vi "Parse RW.vi"(8 "error in (no error)":errorcluster, 11 "R/W mode in":string) -> (0 "error out":errorcluster, 3 "R/W?":T1)   [LabVIEW 2018, in "Config_Read_BML.lvclass"]
uses:
  Config_Read_BML.lvclass
  RW_Option.ctl
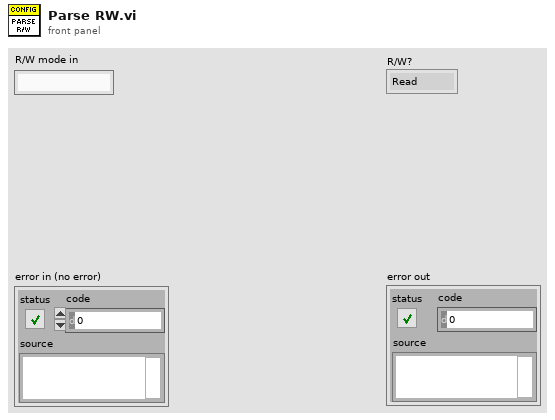
[diagram p1: front panel]
types:
  T1 = typedef "Config_Read_BML.lvclass/RW_Option.ctl" = enum16{"Read", "Write", "R/W"}
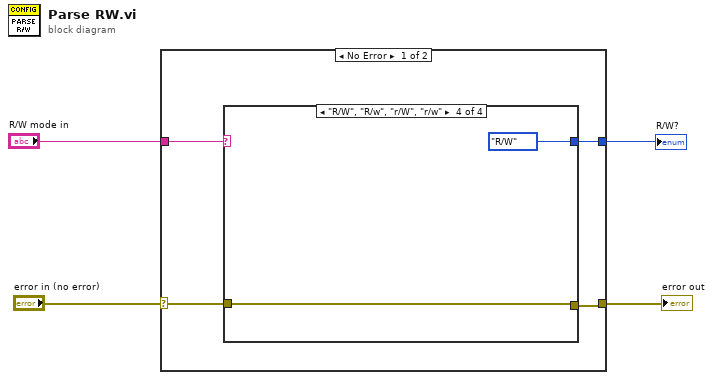
[diagram p0: block diagram]
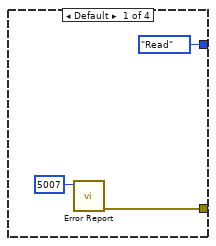
[diagram p2: hidden frame]
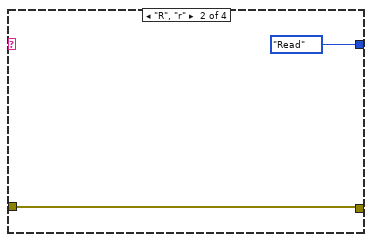
[diagram p3: hidden frame]
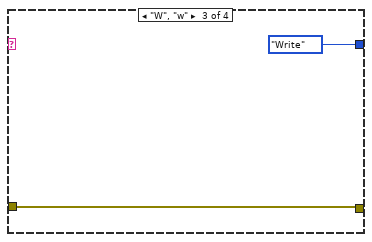
[diagram p4: hidden frame]
diagram:
  n1 = case shown="No Error" "error in (no error)" {
    selector: "error in (no error)" -> [w5 w18]
    tunnel: "R/W mode in" -> [w8 _]
    tunnel: [w6 w18] -> w2
    tunnel: [w7 _] -> w1
    frame No Error {
      n2 = case shown="\"R/W\", \"R/w\", \"r/W\", \"r/w\"" w8 {
        tunnel: [RW_Option."Read" ("R/W?") RW_Option."Read" ("R/W?") RW_Option."Write" ("R/W?") RW_Option."R/W" ("R/W?")] -> w7
        tunnel: [w10 w12 w14 w16] -> w6
        tunnel: w5 -> [_ w12 w14 w16]
        frame Default {
          n3 = call "Error Report.vi"("Error Code"=i16 5007) -> ("error out"=w10:errorcluster)  [unwired: 10 in]
        }
        frame "R", "r" {
        }
        frame "W", "w" {
        }
        frame "R/W", "R/w", "r/W", "r/w" {
        }
      }
    }
    frame Error {
    }
  }
  "error out" <- w2
  "R/W?" <- w1
